vi "Show Spark Status.vi"() -> ()   [LabVIEW 2012]
uses:
  Type/_Log Command.ctl
  Type/_LC Command.ctl
  Configuration/_Global Configuration.vi
panel:
  out "LC Error":string
  out "Vial Pos":string caption="Vial Pos:"
  in  "Read":bool
  out "Detailed Status":string
  out "Plate Pos":string caption="Plate Pos:"
  in  "ClearError":bool
  out "Valve Pos":string caption="Valve Pos:"
  out "Temp":string caption="Temp:"
  out "Status 4":string caption="Status:"
  out "SSV":string caption="SSV:"
  out "ISS":string caption="ISS:"
  out "Tray Temp":string caption="Tray Temp:"
  out "Status 3":string caption="Status:"
  out "Fraction 2":string caption="Fraction:"
  out "Flow 2":string caption="Flow:"
  out "Pressure 2":string caption="Pressure:"
  out "Status 2":string caption="Status:"
  out "Fraction 1":string caption="Fraction:"
  out "Flow 1":string caption="Flow:"
  out "Pressure 1":string caption="Pressure:"
  out "Status 1":string caption="Status:"
  # "Pump 1"
  # "Pump 2"
  # "Bar"
  # "Bar"
  # "ml/min"
  # "ml/min"
  # "%"
  # "%"
  # "Autosampler"
  # "Oven"
  # "deg C"
  # "deg C"
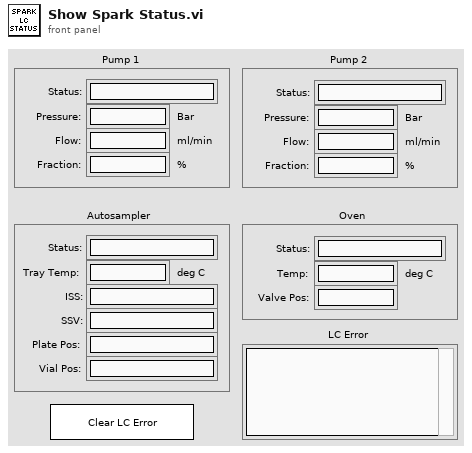
[diagram p1: front panel]
types:
  T1 = typedef "_Log Command.ctl" = enum16{"No Command", "Open", "Read", "Write", "Close", "Check Size"}
  T2 = typedef "_LC Command.ctl" = enum16{"No Command", "Initialize", "Get Configuration", "Get Status", "Get LC Method Contents", "Oven OnOff", "Pump OnOFF", "Rinse Autosampler", "Run Sample", "Set EnvParameters", "Set Method", "Start Equilibration", "Stop Run", "Get LastError", "Clear Error", "Close"}
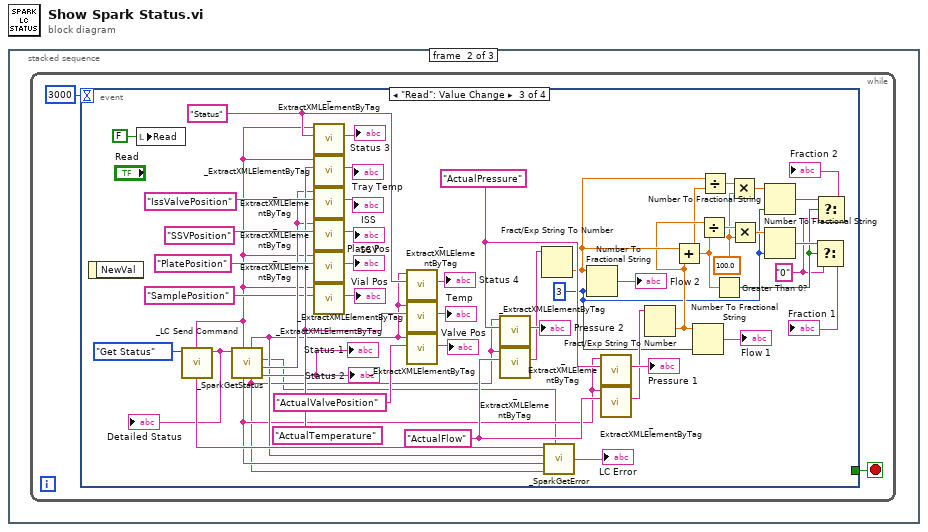
[diagram p0: block diagram]
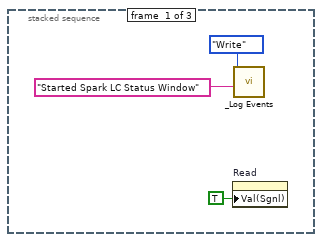
[diagram p2: hidden frame]
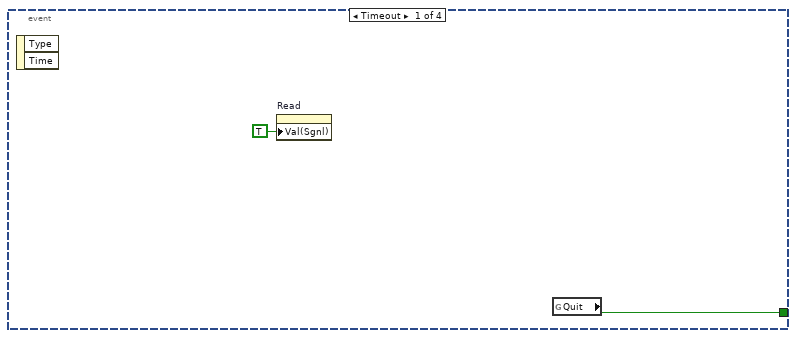
[diagram p3: hidden frame]
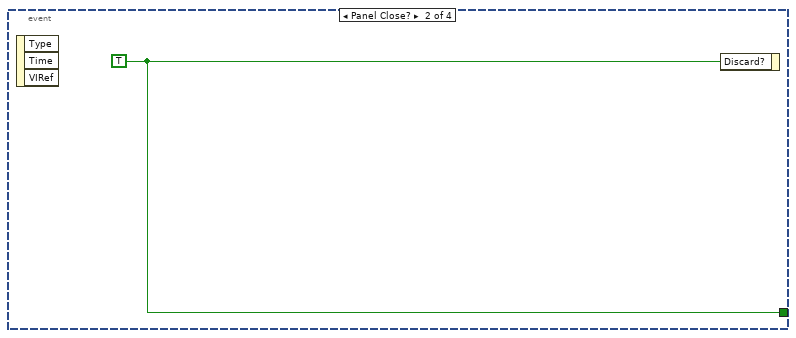
[diagram p4: hidden frame]
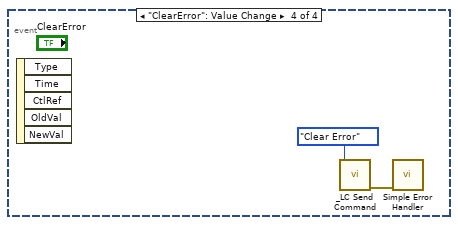
[diagram p5: hidden frame]
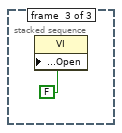
[diagram p6: hidden frame]
diagram:
  n1 = stacked-sequence {
    frame #0 {
      n2 = property on="Read" class="Bool (strict)"("Val(Sgnl)"=TRUE ("Value (Signaling)")) -> ()  [unwired: 2 in, 2 out]
      n3 = call "_Log Events.vi"("Event"="Started Spark LC Status Window" ("string"), "Log Command"=_Log_Command."Write") -> ()  [unwired: 5 in, 2 out]
    }
    frame #1 {
      n4 = while {
        stop <- w4 stop-if-true
        n5 = event shown="[2] \"Read\": Value Change" {
          selector: _ -> [_ _ _ _]
          dyn-events: _ -> [_ _ _ _]
          timeout: 3000 -> [_ _ _ _]
          tunnel: [w7 w8 _ _] -> w4
          event Timeout {
            n6 = event-data() -> ()  [unwired: 1 in, 2 out]
            n7 = property on="Read" class="Bool (strict)"("Val(Sgnl)"=TRUE ("Value (Signaling)")) -> ()  [unwired: 2 in, 2 out]
            n8 = global read "_Global Configuration.vi" "Quit"() -> (w7:bool)
          }
          event Panel Close? {
            w8 = TRUE ("Discard?")
            n9 = event-data() -> ()  [unwired: 1 in, 3 out]
            n10 = event-data("Discard?"=w8) -> ()  [unwired: 1 in, 1 out]
          }
          event "Read": Value Change {
            w16 = "0" ("f")
            w28 = 100.0 ("y")
            w25 = i16 3 ("precision (6)")
            w50 = "ActualTemperature"
            w54 = "ActualPressure"
            w53 = "ActualFlow"
            w56 = "Status"
            n11 = event-data() -> ()  [unwired: 1 in, 1 out]
            n12 = local write "Read"(FALSE ("Read")) -> ()
            n13 = call "_LC Send Command.vi"("Command"=_LC_Command."Get Status") -> ("Reply"=w10:string)  [unwired: 9 in, 1 out]
            "Detailed Status" <- w10
            n14 = call "_SparkGetStatus.vi"("SparkStatus"=w10) -> ("PumpState"=→"Status 1" →"Status 2":string, "AS Status 2"=w38:string, "LCStatus"=w9:string, "PumpB Status"=w11:string, "Oven Status"=w13:string, "PumpA Status"=w12:string, "AS Status"=w14:string)  [unwired: 3 in, 1 out]
            n15 = call "_ExtractXMLElementByTag.vi"("TagName"=w56, "XML String"=w14) -> ("Element"=→"Status 3":string)  [unwired: 2 in, 3 out]
            n16 = call "_ExtractXMLElementByTag.vi"("TagName"=w50, "XML String"=w14) -> ("Element"=→"Tray Temp":string)  [unwired: 2 in, 3 out]
            n17 = call "_ExtractXMLElementByTag.vi"("TagName"="IssValvePosition", "XML String"=w38) -> ("Element"=→"ISS":string)  [unwired: 2 in, 3 out]
            n18 = call "_ExtractXMLElementByTag.vi"("TagName"="SSVPosition", "XML String"=w38) -> ("Element"=→"SSV":string)  [unwired: 2 in, 3 out]
            n19 = call "_ExtractXMLElementByTag.vi"("TagName"="PlatePosition", "XML String"=w14) -> ("Element"=→"Plate Pos":string)  [unwired: 2 in, 3 out]
            n20 = call "_ExtractXMLElementByTag.vi"("TagName"="SamplePosition", "XML String"=w14) -> ("Element"=→"Vial Pos":string)  [unwired: 2 in, 3 out]
            n21 = call "_ExtractXMLElementByTag.vi"("TagName"=w56, "XML String"=w13) -> ("Element"=→"Status 4":string)  [unwired: 2 in, 3 out]
            n22 = call "_ExtractXMLElementByTag.vi"("TagName"=w50, "XML String"=w13) -> ("Element"=→"Temp":string)  [unwired: 2 in, 3 out]
            n23 = call "_ExtractXMLElementByTag.vi"("TagName"="ActualValvePosition", "XML String"=w13) -> ("Element"=→"Valve Pos":string)  [unwired: 2 in, 3 out]
            n24 = call "_ExtractXMLElementByTag.vi"("TagName"=w54, "XML String"=w11) -> ("Element"=→"Pressure 2":string)  [unwired: 2 in, 3 out]
            n25 = call "_ExtractXMLElementByTag.vi"("TagName"=w53, "XML String"=w11) -> ("Element"=w36:string)  [unwired: 2 in, 3 out]
            n26 = Fract/Exp String To Number(string=w36) -> (number=w32:dbl)  [unwired: 3 in, 1 out]
            n27 = call "_SparkGetError.vi"("AS Status"=w14, "Oven Status"=w13, "Pump 1 Status"=w12, "Pump 2 Status"=w11, "LC Status"=w9) -> ("LC Error"=→"LC Error":string)
            n28 = Number To Fractional String(number=w32, precision (6)=w25) -> (F-format string=→"Flow 2":string)  [unwired: 2 in]
            n29 = call "_ExtractXMLElementByTag.vi"("TagName"=w54, "XML String"=w12) -> ("Element"=→"Pressure 1":string)  [unwired: 2 in, 3 out]
            n30 = call "_ExtractXMLElementByTag.vi"("TagName"=w53, "XML String"=w12) -> ("Element"=w35:string)  [unwired: 2 in, 3 out]
            n31 = Fract/Exp String To Number(string=w35) -> (number=w31:dbl)  [unwired: 3 in, 1 out]
            n32 = Add(x=w32, y=w31) -> (x+y=w22:dbl)
            n33 = Number To Fractional String(number=w31, precision (6)=w25) -> (F-format string=→"Flow 1":string)  [unwired: 2 in]
            n34 = Divide(x=w31, y=w22) -> (x/y=w29:dbl)
            n35 = Divide(x=w32, y=w22) -> (x/y=w30:dbl)
            n36 = Greater Than 0?(x=w22) -> (x > 0?=w19:bool)
            n37 = Multiply(x=w30, y=w28) -> (x*y=w27:dbl)
            n38 = Multiply(x=w29, y=w28) -> (x*y=w26:dbl)
            n39 = Number To Fractional String(number=w27, precision (6)=w25) -> (F-format string=w21:string)  [unwired: 2 in]
            n40 = Number To Fractional String(number=w26, precision (6)=w25) -> (F-format string=w20:string)  [unwired: 2 in]
            n41 = Select(t=w20, s=w19, f=w16) -> (s? t:f=→"Fraction 1":string)
            n42 = Select(t=w21, s=w19, f=w16) -> (s? t:f=→"Fraction 2":string)
          }
          event "ClearError": Value Change {
            n43 = event-data() -> ()  [unwired: 1 in, 5 out]
            n44 = call "_LC Send Command.vi"("Command"=_LC_Command."Clear Error") -> ("error out"=w59:errorcluster)  [unwired: 9 in, 1 out]
            n45 = call <vilib>:"Simple Error Handler.vi"("error in (no error)"=w59) -> ()  [unwired: 4 in, 5 out]
          }
        }
      }
    }
    frame #2 {
      n46 = property class="VI"("Front Panel.Open"=FALSE ("Front Panel Window:Open")) -> ()  [unwired: 2 in, 2 out]
    }
  }
